vi "Control de un motor en arduino con un PWM.vi"() -> ()   [LabVIEW 2020]
doc: "Este VI controla un motor fisico conectado en Arduino a través de una señal PWM, modifica la velocidad del motor y su dirección."
uses:
  <vilib>/MakerHub/LINX/Public/Peripherals/Digital/Digital Write 1 Chan.vi
  <vilib>/MakerHub/LINX/Public/Peripherals/Digital/Digital Write N Chans.vi
  <vilib>/MakerHub/LINX/Private/Local IO/LinxDigitalWrite.vi
  <vilib>/MakerHub/LINX/Public/Utilities/Check Channel.vi
  <vilib>/MakerHub/LINX/Public/Utilities/Open Serial.vi
  <vilib>/MakerHub/LINX/Private/Utilties/Generate Error.vi
  <vilib>/MakerHub/LINX/LMH-LINX.lvlib
panel:
  in  "stop":bool
  out "Señal PWM":dbl(graph)
  out "Elapsed Time (s)":dbl
  in  "Duty cicle":dbl(knob) scale=0.0..100.0
  in  "Frequency":dbl(knob) scale=0.0..10.0
  in  "Direccion motor":bool
  in  "Serial Port":refnum<visa-resource-name>="N/A"
  in  "Motor Direction Pin 2":u8
  in  "Motor Direction Pin 1":u8
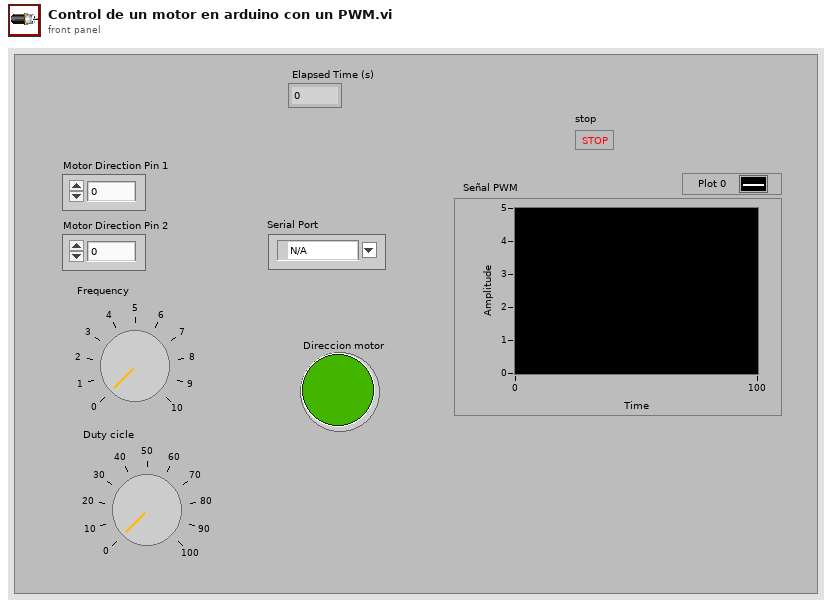
[diagram p1: front panel]
types:
  T1 = typedef "LMH-LINX.lvlib/LINX Ref.ctl" = cluster{"IO":T2, "Interface":T3, "LINX Device Config":T4}
  T2 = typedef "LMH-LINX.lvlib/Platform.ctl" = enum16{"Remote", "Local"}
  T3 = typedef "LMH-LINX.lvlib/Interface.ctl" = enum16{"Serial", "TCP"}
  T4 = typedef "LMH-LINX.lvlib/Device.lvlib/LINX Device Config.ctl" = cluster{"Interface":T3, "COM Port":refnum<visa-resource-name>, "TCP Configuration":T5, "Device Family":u8, "Device ID":u8, "Device Name":string, "TCP Ref":refnum<k5>, "Channels":T6}
  T5 = typedef "LMH-LINX.lvlib/Device.lvlib/TCP Config.ctl" = cluster{"IP Address":string, "Port":u16}
  T6 = typedef "LMH-LINX.lvlib/Channels.ctl" = cluster{"DI":u8[], "DO":u8[], "AI":u8[], "AO":u8[], "PWM":u8[], "QE":u8[], "UART":u8[], "I2C 2":u8[], "SPI":u8[], "CAN":u8[], "Servo":u8[], "AI Ref (V)":dbl, "AI Resolution (Bits)":u8, "AO Ref (V)":dbl, "AO Resolution (Bits)":u8}
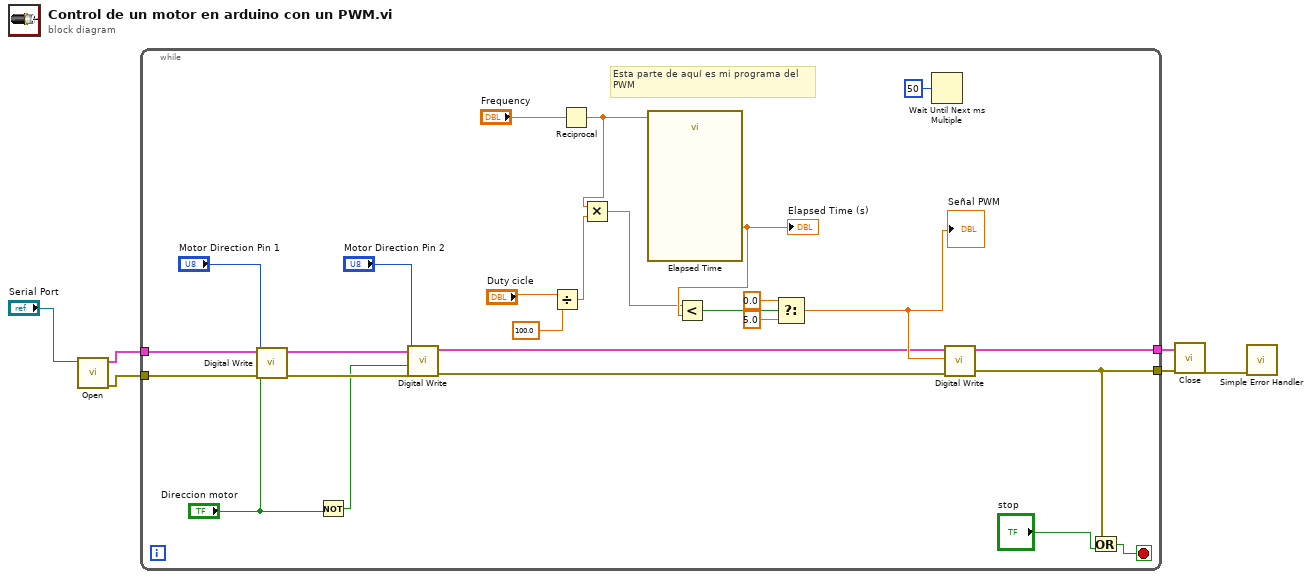
[diagram p0: block diagram]
diagram:
  n1 = call-poly <vilib>:"Open.vi"("Serial Port"="Serial Port") -> ("Error Out"=w5:errorcluster, "LINX Resource"=w6:T1)  [unwired: 8 in, 1 out]
  n2 = while {
    tunnel: w6 -> [w32]
    tunnel: w5 -> [w31]
    tunnel: [w7] -> w2
    tunnel: [w12] -> w1
    stop <- w9 stop-if-true
    # "Esta parte de aquí es mi programa del \nPWM"
    n3 = call-poly <vilib>:"Digital Write.vi"("Error In"=w31, "Output Value"="Direccion motor", "DO Channel"="Motor Direction Pin 1", "LINX Resource"=w32) -> ("Error Out"=w30:errorcluster, "LINX Resource"=w29:T1)  [unwired: 6 in]
    n4 = Not(x="Direccion motor") -> (.not. x?=w25:bool)
    n5 = call-poly <vilib>:"Digital Write.vi"("Error In"=w30, "Output Value"=w25, "DO Channel"="Motor Direction Pin 2", "LINX Resource"=w29) -> ("Error Out"=w13:errorcluster, "LINX Resource"=w10:T1)  [unwired: 6 in]
    n6 = Divide(x="Duty cicle", y=100.0) -> (x/y=w20:dbl)
    n7 = Reciprocal(x="Frequency") -> (1/x=w19:dbl)
    n8 = Multiply(x=w19, y=w20) -> (x*y=w14:dbl)
    n9 = call "Elapsed Time"("Time Target (s)"=w19) -> ("Elapsed Time (s)"=w15:dbl)  [unwired: 11 in, 7 out]
    "Elapsed Time (s)" <- w15
    n10 = Less?(x=w14, y=w15) -> (x < y?=w18:bool)
    n11 = Select(t=0.0, s=w18, f=5.0) -> (s? t:f=w11:dbl)
    "Señal PWM" <- w11
    n12 = Wait Until Next ms Multiple(millisecond multiple=u32 50) -> ()  [unwired: 1 out]
    n13 = call-poly <vilib>:"Digital Write.vi"("Error In"=w13, "DO Channel"=w11, "LINX Resource"=w10) -> ("Error Out"=w7:errorcluster, "LINX Resource"=w12:T1)  [unwired: 7 in]
    n14 = Or(x=w7, y="stop") -> (x .or. y?=w9:bool)
  }
  n15 = call <vilib>:"Close.vi"("Error In"=w2, "LINX Resource"=w1) -> ("Error Out"=w4:errorcluster)  [unwired: 9 in]
  n16 = call <vilib>:"Simple Error Handler.vi"("error in (no error)"=w4) -> ()  [unwired: 4 in, 5 out]
